vi "HEADERS Request.vi"(7 "Header":T1, 8 "error in (no error)":errorcluster, 9 "Single Header Name":string, 10 "Path (after URL)":string, 11 "EnVision REST in":refnum<class "EnVision REST.lvclass">) -> (0 "error out":errorcluster, 1 "Header Value(s)":string[](array[string]), 2 "Header Name(s)":string[](array[string]), 3 "EnVision REST out":refnum<class "EnVision REST.lvclass">, 4 "Status Code":u16)   [LabVIEW 2018, in "EnVision REST.lvlib" / "EnVision REST.lvclass"]
uses:
  EnVision REST.lvclass
  PPLs/REST Interface/Parent/REST Interface.lvlibp/Custom Controls/Headers.ctl
  EnVision REST.lvclass/EnVision REST.ctl
  <vilib>/addons/_JKI.lib/REST Client/classes/REST Client/REST Client.lvclass
  <vilib>/addons/_JKI.lib/REST Client/classes/Response Headers/Response Headers.lvclass
  PPLs/REST Interface/Parent/REST Interface.lvlibp/REST Interface.lvclass
  C:/Projects/LabVIEW/PPLs/REST Interface/Parent/REST Interface.lvlibp/REST Interface.lvclass
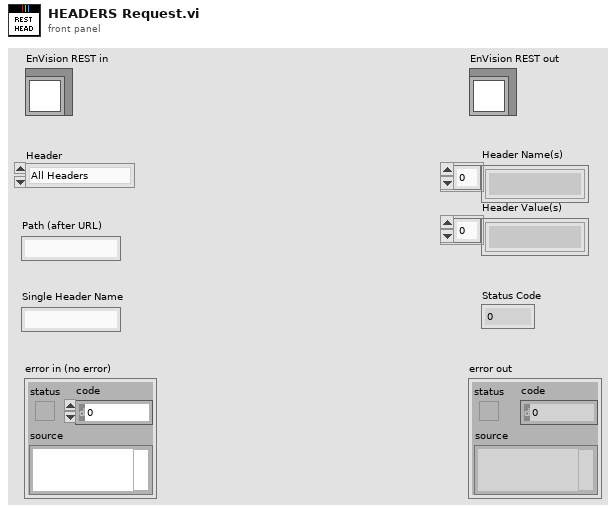
[diagram p1: front panel]
types:
  T1 = typedef "REST Interface.lvlibp/REST Interface.lvclass/Headers.ctl" = enum16{"All Headers", "Single Header"}
  T2 = typedef "REST Interface.lvlibp/REST Client.lvlib/REST Client.lvclass/HTTP Header.ctl" = cluster{"header":string, "value":string}
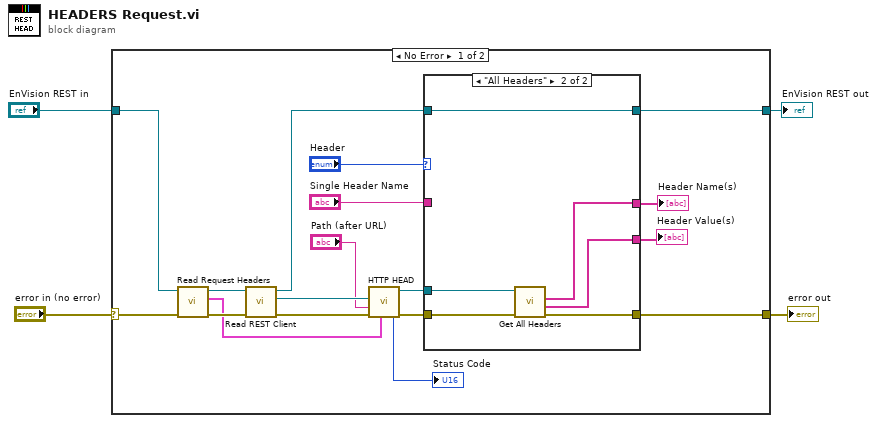
[diagram p0: block diagram]
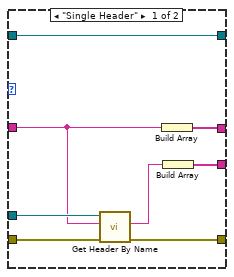
[diagram p2: hidden frame]
diagram:
  n1 = case shown="No Error" "error in (no error)" {
    selector: "error in (no error)" -> [w8 w38]
    tunnel: [w12 w38] -> w3
    tunnel: [w22 w37] -> w2
    tunnel: "EnVision REST in" -> [w9 w37]
    frame No Error {
      n2 = call "Read Request Headers.vi"("error in (no error)"=w8, "REST Interface in"=w9) -> ("error out"=w7:errorcluster, "Request Headers"=w5:T2[], "REST Interface out"=w6:refnum<class "EnVision REST.lvclass">)  [unwired: 7 in]
      n3 = call "Read REST Client.vi"("error in (no error)"=w7, "EnVision REST in"=w6) -> ("error out"=w17:errorcluster, "REST Client.lvlib:REST Client.lvclass"=w18:refnum<class "REST Client.lvclass">, "EnVision REST out"=w21:refnum<class "EnVision REST.lvclass">)  [unwired: 7 in]
      n4 = call-dynamic "HTTP HEAD.vi"("request specific headers"=w5, "error in (no error)"=w17, "Path"="Path (after URL)", "REST Client in"=w18) -> ("error out"=w15:errorcluster, "Response Headers"=w16:refnum<class "Response Headers.lvclass">, "Status Code"=→"Status Code":u16)  [unwired: 2 in, 3 out]
      n5 = case shown="\"All Headers\"" "Header" {
        tunnel: [w30 w36] -> w22
        tunnel: w21 -> [w30 w36]
        tunnel: "Single Header Name" -> [w27 _]
        tunnel: w16 -> [w28 w34]
        tunnel: w15 -> [w29 w35]
        tunnel: [w26 w32] -> w14
        tunnel: [w24 w31] -> w13
        tunnel: [w23 w33] -> w12
        frame "Single Header" {
          n6 = call <vilib>:"Get Header By Name.vi"("error in (no error)"=w29, "Name"=w27, "Response Headers in"=w28) -> ("error out"=w23:errorcluster, "Value"=w25:string)  [unwired: 5 in, 2 out]
          n7 = Build Array(w27) -> (w26:string[])
          n8 = Build Array(w25) -> (w24:string[])
        }
        frame "All Headers" {
          n9 = call <vilib>:"Get All Headers.vi"("error in (no error)"=w35, "Response Headers in"=w34) -> ("error out"=w33:errorcluster, "Values"=w31:string[], "Names"=w32:string[])  [unwired: 6 in, 1 out]
        }
      }
      "Header Value(s)" <- w13
      "Header Name(s)" <- w14
    }
    frame Error {
    }
  }
  "error out" <- w3
  "EnVision REST out" <- w2
